vi "Pump Set Volume.vi"(8 "error in (no error)":errorcluster, 10 "Target Volume (ul)":i32, 11 "Application in":refnum<class "Application.lvclass">) -> (0 "error out":errorcluster, 3 "Application out":refnum<class "Application.lvclass">)   [LabVIEW 2015, in "Application.lvlib" / "Application.lvclass"]
uses:
  Application.lvclass
  Application.lvclass/Application.ctl
  Hardware/PHD Ultra Messages/Set Volume Msg/Set Volume Msg.lvclass/Set Volume Msg.ctl
  <vilib>/ActorFramework/Message Enqueuer/Message Enqueuer.lvclass/Message Enqueuer.ctl
  <vilib>/ActorFramework/Message Enqueuer/Enqueue.vi
  <vilib>/ActorFramework/Message Priority Queue/Priority Enqueue.vi
  Hardware/PHD Ultra Messages/Set Volume Msg/Set Volume Msg.lvclass
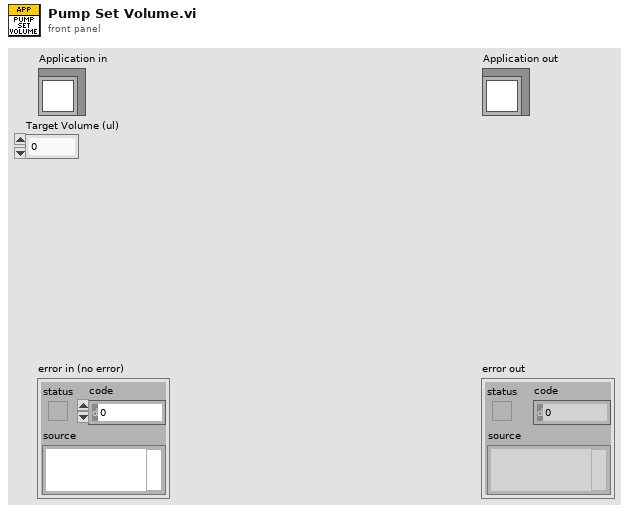
[diagram p1: front panel]
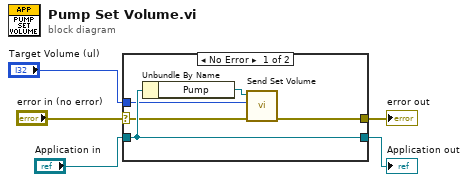
[diagram p0: block diagram]
diagram:
  n1 = case shown="No Error" "error in (no error)" {
    selector: "error in (no error)" -> [w8 w12]
    tunnel: [w7 w12] -> w4
    tunnel: [w10 w11] -> w2
    tunnel: "Application in" -> [w10 w11]
    tunnel: "Target Volume (ul)" -> [w6 _]
    frame No Error {
      n2 = Unbundle By Name(w10) -> ("Pump"=w9:refnum<class "Message Enqueuer.lvclass">)
      n3 = call "Send Set Volume.vi"("error in (no error)"=w8, "Target Volume (ul)"=w6, "Message Enqueuer"=w9) -> ("error out"=w7:errorcluster)  [unwired: 7 in, 1 out]
    }
    frame Error {
    }
  }
  "error out" <- w4
  "Application out" <- w2
